vi "remove_invalid_ROI.vi"(8 "error in (no error)":errorcluster, 9 "number of particles":i32, 10 "neighborhood array":T1[](array[typedef]), 11 "Image Pixels in":u8[][](array[numeric])) -> (0 "error out":errorcluster, 2 "ROI array out":T1[](array[typedef]), 3 "Image Pixels out":u8[][](array[numeric]))   [LabVIEW 2010]
uses:
  point_cluster.ctl
panel:
  out "Numeric":i32
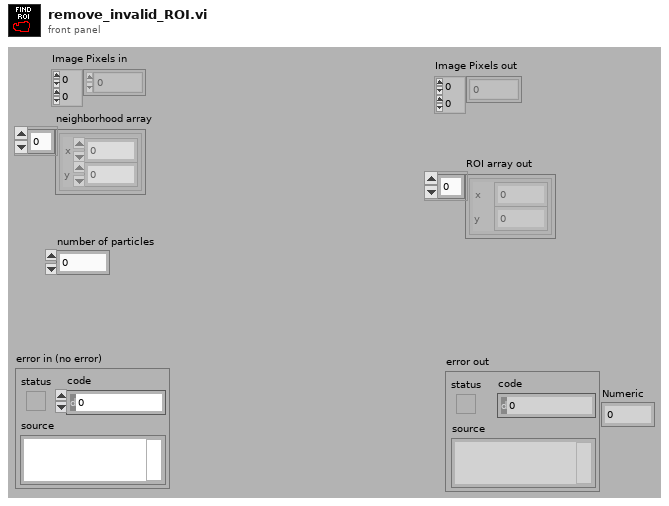
[diagram p1: front panel]
types:
  T1 = typedef "point_cluster.ctl" = cluster{"x":i32, "y":i32}
  T2 = cluster{"[0]":i32, "[1]":i32, "[2]":i32, "[3]":i32, "[4]":i32, "[5]":i32, "[6]":i32, "[7]":i32, "[8]":i32}
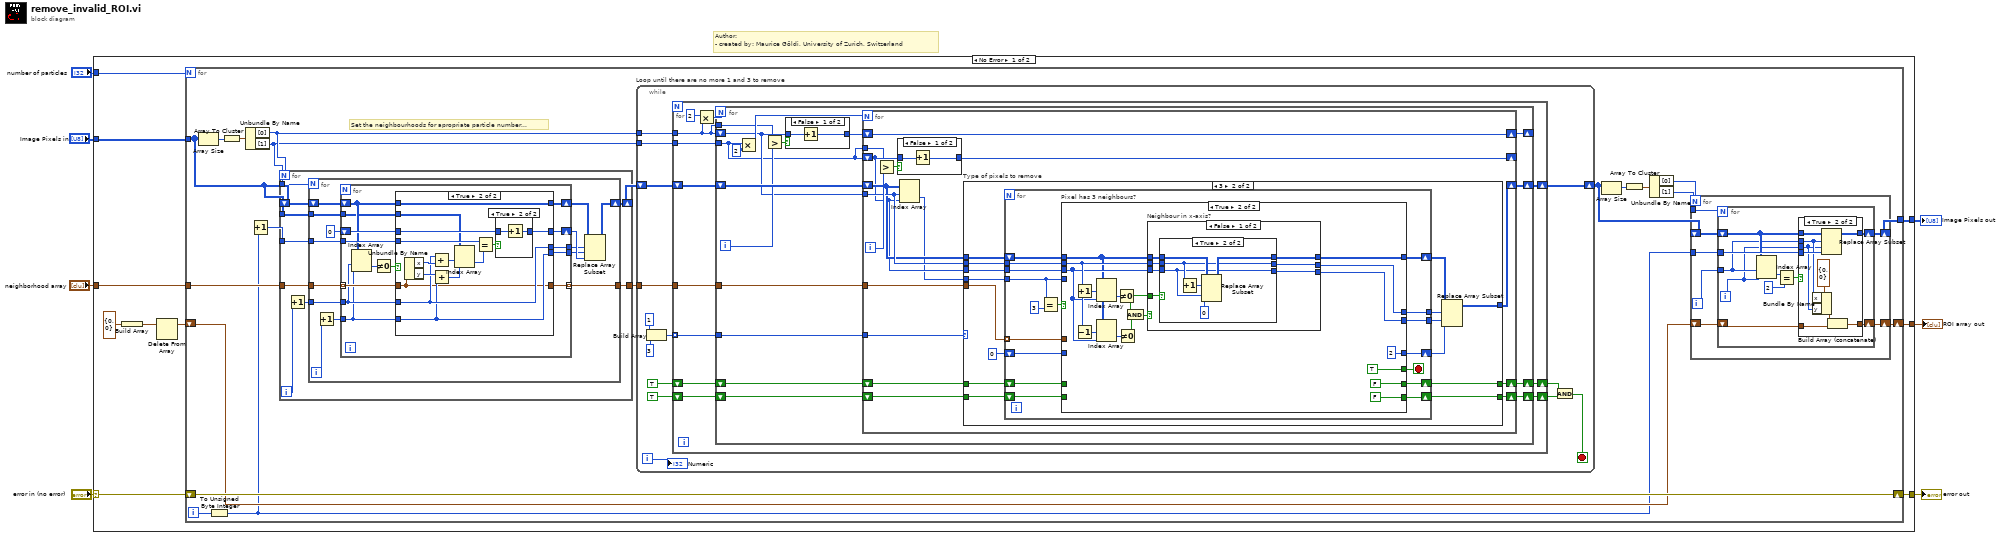
[diagram p0: block diagram]
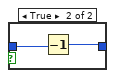
[diagram p5: hidden frame]
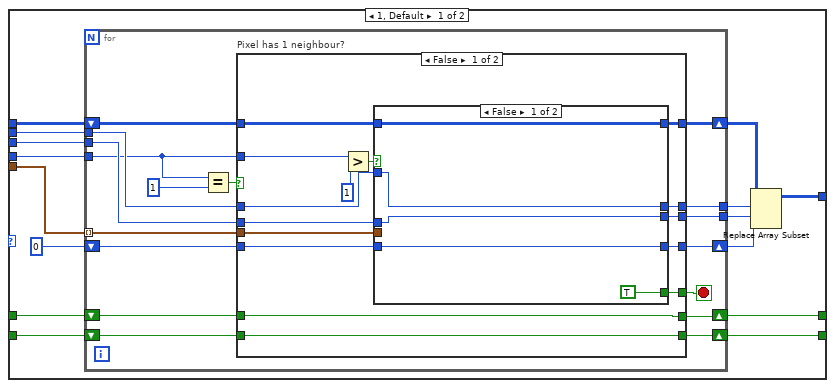
[diagram p6: hidden frame]
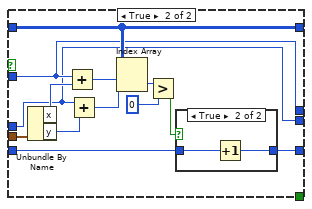
[diagram p7: hidden frame]
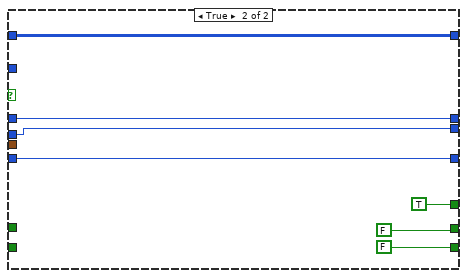
[diagram p9: hidden frame]
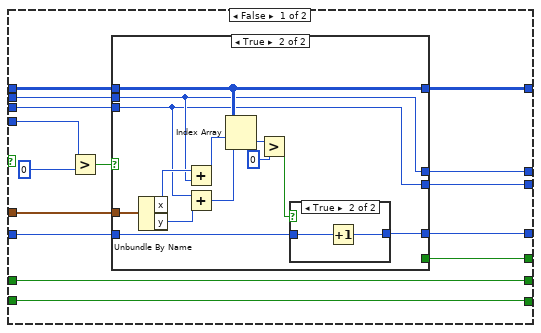
[diagram p10: hidden frame]
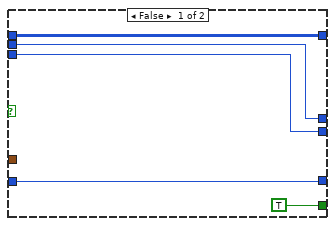
[diagram p11: hidden frame]
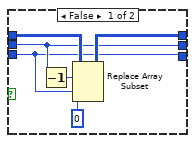
[diagram p13: hidden frame]
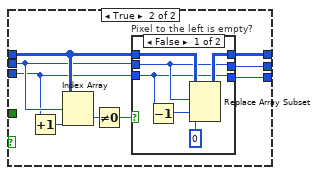
[diagram p14: hidden frame]
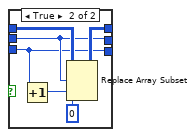
[diagram p15: hidden frame]
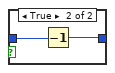
[diagram p16: hidden frame]
diagram:
  # "Author: \n- created by: Maurice Göldi, University of Zurich, Switzerland"
  n1 = case shown="No Error" "error in (no error)" {
    selector: "error in (no error)" -> [w14 w392]
    tunnel: [w13 w392] -> w6
    tunnel: "number of particles" -> [w17 _]
    tunnel: "Image Pixels in" -> [w16 _]
    tunnel: "neighborhood array" -> [w15 _]
    tunnel: [w12 _] -> w2
    tunnel: [w11 _] -> w1
    frame No Error {
      n2 = Build Array(T1 {"x"=0, "y"=0} ("point")) -> (w9:T1[])
      n3 = Delete From Array(array=w9) -> (array with subset deleted=w8:T1[])  [unwired: 2 in, 1 out]
      n4 = for {
        N: w17 -> [_]
        tunnel: w16 -> [w18]
        tunnel: w15 -> [w32]
        shift-right: [w37] -> w13
        shift-left: w14 -> [w37]
        shift-right: [w25] -> w12
        shift-left: w8 -> [w24]
        tunnel: [w23] -> w11
        i -> [w22]
        # "Set the neighbourhoods for apropriate particle number..."
        n5 = Array Size(array=w18) -> (size(s)=w36:i32[])
        n6 = To Unsigned Byte Integer(number=w22) -> (unsigned 8bit integer=w21:u8)
        n7 = Array To Cluster(array=w36) -> (cluster=w35:T2)
        n8 = Unbundle By Name(w35) -> ("[0]"=w34:i32, "[1]"=w33:i32)
        n9 = Increment(x=w21) -> (x+1=w30:u8)
        n10 = for {
          N: w34 -> [_]
          tunnel: w33 -> [w74]
          shift-right: [w72] -> w20
          shift-left: w18 -> [w73]
          tunnel: w32 -> [w71]
          tunnel: [w70] -> w31
          tunnel: w30 -> [w67]
          tunnel: w18 -> [w66]
          i -> [w69]
          n11 = Increment(x=w69) -> (x+1=w68:i32)
          n12 = for {
            N: w74 -> [_]
            shift-right: [w79] -> w72
            shift-left: w73 -> [w86]
            tunnel: [w88] -> w70
            tunnel: w71 -> [w87]
            tunnel: w68 -> [w84]
            tunnel: w67 -> [w82]
            tunnel: w66 -> [w75]
            i -> [w85]
            n13 = Increment(x=w85) -> (x+1=w83:i32)
            n14 = for {
              tunnel: [w90] -> w88 mode=indexing
              tunnel: w87 -> [w102] mode=indexing
              shift-right: [w97] -> w80
              shift-left: w86 -> [w95]
              tunnel: w84 -> [w94]
              tunnel: w83 -> [w93]
              tunnel: w82 -> [w96]
              shift-right: [w100] -> w78
              shift-left: u8 0 -> [w101]
              tunnel: [w99] -> w77
              tunnel: [w98] -> w76
              tunnel: w75 -> [w89]
              n15 = Index Array(array=w95, index (row)=w94, index (col)=w93) -> (element=w91:u8)
              n16 = Not Equal To 0?(x=w91) -> (x != 0?=w92:bool)
              n17 = case shown="True" w92 {
                tunnel: w102 -> [w103 w109]
                tunnel: w95 -> [w104 w110]
                tunnel: w96 -> [_ w115]
                tunnel: w101 -> [w105 w114]
                tunnel: [w105 w113] -> w100
                tunnel: w93 -> [w106 w111]
                tunnel: w94 -> [w107 w112]
                tunnel: [w107 w112] -> w99
                tunnel: [w106 w111] -> w98
                tunnel: [w104 w110] -> w97
                tunnel: [w103 w109] -> w90
                tunnel: w89 -> [_ w108]
                frame False {
                }
                frame True {
                  n18 = Unbundle By Name(w109) -> ("x"=w121:i32, "y"=w120:i32)
                  n19 = Add(x=w112, y=w121) -> (x+y=w119:i32)
                  n20 = Add(x=w120, y=w111) -> (x+y=w118:i32)
                  n21 = Index Array(array=w108, index (row)=w119, index (col)=w118) -> (element=w116:u8)
                  n22 = Equal?(x=w115, y=w116) -> (x = y?=w117:bool)
                  n23 = case shown="True" w117 {
                    tunnel: [w122 w124] -> w113
                    tunnel: w114 -> [w122 w123]
                    frame False {
                    }
                    frame True {
                      n24 = Increment(x=w123) -> (x+1=w124:u8)
                    }
                  }
                }
              }
            }
            n25 = Replace Array Subset(array=w80, new element=w78, index (row)=w77, index (col)=w76) -> (w79:u8[][])
          }
        }
        n26 = while "Loop until there are no more 1 and 3 to remove" {
          tunnel: w31 -> [w138]
          tunnel: w34 -> [w133]
          tunnel: w33 -> [w132]
          shift-right: [w131] -> w19
          shift-left: w20 -> [w130]
          i -> [w129]
          stop <- w127 stop-if-true
          n27 = Build Array(1 ("element"), 3 ("element")) -> (w135:i32[])
          n28 = for {
            tunnel: w138 -> [w147]
            tunnel: w135 -> [w146] mode=indexing
            tunnel: w133 -> [w142]
            tunnel: w132 -> [w144]
            shift-right: [w143] -> w131
            shift-left: w130 -> [w150]
            shift-right: [w139] -> w126
            shift-left: TRUE -> [w145]
            shift-right: [w140] -> w125
            shift-left: TRUE -> [w141]
            n29 = Multiply(x=2, y=w142) -> (x*y=w149:i32)
            n30 = for {
              N: w149 -> [_]
              tunnel: w144 -> [w153]
              shift-right: [w165] -> _
              shift-left: w142 -> [w159]
              shift-right: [w163] -> w143
              shift-left: w150 -> [w164]
              tunnel: w147 -> [w158]
              tunnel: w146 -> [w157]
              shift-right: [w155] -> w139
              shift-left: w145 -> [w156]
              tunnel: w142 -> [w154]
              shift-right: [w151] -> w140
              shift-left: w141 -> [w152]
              i -> [w160]
              n31 = Multiply(x=w153, y=2) -> (x*y=w166:i32)
              n32 = Greater?(x=w154, y=w160) -> (0:w161:bool)
              n33 = case shown="False" w161 {
                tunnel: w159 -> [w169 w170]
                tunnel: [w168 w171] -> w162
                frame False {
                  n34 = Increment(x=w169) -> (x+1=w168:i32)
                }
                frame True {
                  n35 = Decrement(x=w170) -> (x-1=w171:i32)
                }
              }
              n36 = for {
                N: w166 -> [_]
                shift-right: [w187] -> w165
                shift-left: w162 -> [w187]
                shift-right: [w186] -> _
                shift-left: w153 -> [w179]
                shift-right: [w177] -> w163
                shift-left: w164 -> [w180]
                tunnel: w159 -> [w181]
                tunnel: w158 -> [w183]
                tunnel: w157 -> [w182]
                shift-right: [w175] -> w155
                shift-left: w156 -> [w176]
                tunnel: w153 -> [w174]
                shift-right: [w172] -> w151
                shift-left: w152 -> [w173]
                i -> [w184]
                n37 = Greater?(x=w174, y=w184) -> (0:w185:bool)
                n38 = case shown="False" w185 {
                  tunnel: w179 -> [w389 w390]
                  tunnel: [w388 w391] -> w186
                  frame False {
                    n39 = Increment(x=w389) -> (x+1=w388:i32)
                  }
                  frame True {
                    n40 = Decrement(x=w390) -> (x-1=w391:i32)
                  }
                }
                n41 = Index Array(array=w180, index (row)=w181, index (col)=w179) -> (element=w178:u8)
                n42 = case "Type of pixels to remove" shown="3" w182 {
                  tunnel: w183 -> [w202 w273]
                  tunnel: w181 -> [w201 w276]
                  tunnel: w179 -> [w200 w275]
                  tunnel: w180 -> [w199 w277]
                  tunnel: w178 -> [w198 w274]
                  tunnel: [w192 w271] -> w177
                  tunnel: w176 -> [w190 w267]
                  tunnel: [w189 w266] -> w175
                  tunnel: w173 -> [w191 w264]
                  tunnel: [w188 w263] -> w172
                  frame 1, Default {
                    n43 = for {
                      tunnel: w202 -> [w213] mode=indexing
                      tunnel: w201 -> [w217]
                      tunnel: w200 -> [w216]
                      shift-right: [w210] -> w195
                      shift-left: w199 -> [w214]
                      tunnel: w198 -> [w215]
                      shift-right: [w211] -> w196
                      shift-left: u8 0 -> [w212]
                      tunnel: [w209] -> w194
                      tunnel: [w208] -> w193
                      shift-right: [w206] -> w188
                      shift-left: w191 -> [w205]
                      shift-right: [w203] -> w189
                      shift-left: w190 -> [w204]
                      stop <- w207 stop-if-true
                      n44 = Equal?(x=w215, y=u8 1) -> (x = y?=w218:bool)
                      n45 = case "Pixel has 1 neighbour?" shown="False" w218 {
                        tunnel: w214 -> [w226 w261]
                        tunnel: w217 -> [w230 w260]
                        tunnel: w216 -> [w229 w259]
                        tunnel: w215 -> [w233 _]
                        tunnel: w213 -> [w231 _]
                        tunnel: w212 -> [w228 w262]
                        tunnel: [w227 w262] -> w211
                        tunnel: [w225 w261] -> w210
                        tunnel: [w224 w260] -> w209
                        tunnel: [w223 w259] -> w208
                        tunnel: [w222 TRUE] -> w207
                        tunnel: [w220 FALSE] -> w206
                        tunnel: w205 -> [w220 _]
                        tunnel: [w221 FALSE] -> w203
                        tunnel: w204 -> [w221 _]
                        frame False {
                          n46 = Greater?(x=w233, y=u8 1) -> (0:w234:bool)
                          n47 = case shown="False" w234 {
                            tunnel: w226 -> [w238 w244]
                            tunnel: w231 -> [_ w250]
                            tunnel: w230 -> [w237 w243]
                            tunnel: w229 -> [w236 w242]
                            tunnel: w228 -> [w239 w246]
                            tunnel: [w239 w245] -> w227
                            tunnel: [w238 w244] -> w225
                            tunnel: [w237 w243] -> w224
                            tunnel: [w236 w242] -> w223
                            tunnel: [TRUE _] -> w222
                            frame False {
                            }
                            frame True {
                              n48 = Unbundle By Name(w250) -> ("x"=w251:i32, "y"=w252:i32)
                              n49 = Add(x=w243, y=w251) -> (x+y=w241:i32)
                              n50 = Add(x=w242, y=w252) -> (x+y=w240:i32)
                              n51 = Index Array(array=w244, index (row)=w241, index (col)=w240) -> (element=w249:u8)
                              n52 = Greater?(x=w249, y=u8 0) -> (0:w247:bool)
                              n53 = case shown="True" w247 {
                                tunnel: w246 -> [w253 w255]
                                tunnel: [w253 w254] -> w245
                                frame False {
                                }
                                frame True {
                                n54 = Increment(x=w255) -> (x+1=w254:u8)
                                }
                              }
                            }
                          }
                        }
                        frame True {
                        }
                      }
                    }
                    n55 = Replace Array Subset(array=w195, new element=w196, index (row)=w194, index (col)=w193) -> (w192:u8[][])
                  }
                  frame 3 {
                    n56 = for {
                      tunnel: w276 -> [w291]
                      tunnel: w275 -> [w290]
                      tunnel: w274 -> [w282]
                      tunnel: w273 -> [w289] mode=indexing
                      shift-right: [w286] -> w265
                      shift-left: w277 -> [w294]
                      shift-right: [w287] -> w268
                      shift-left: u8 0 -> [w288]
                      tunnel: [w285] -> w270
                      tunnel: [w284] -> w269
                      shift-right: [w280] -> w266
                      shift-left: w267 -> [w281]
                      shift-right: [w278] -> w263
                      shift-left: w264 -> [w279]
                      stop <- w283 stop-if-true
                      n57 = Equal?(x=w282, y=u8 3) -> (x = y?=w293:bool)
                      n58 = case "Pixel has 3 neighbours?" shown="True" w293 {
                        tunnel: w294 -> [w307 w336]
                        tunnel: w291 -> [w305 w338]
                        tunnel: w290 -> [w304 w337]
                        tunnel: w289 -> [w306 _]
                        tunnel: w288 -> [w308 _]
                        tunnel: [w309 u8 2] -> w287
                        tunnel: [w303 w335] -> w286
                        tunnel: [w302 w332] -> w285
                        tunnel: [w301 w331] -> w284
                        tunnel: [w297 TRUE] -> w283
                        tunnel: w282 -> [w298 _]
                        tunnel: w281 -> [w295 _]
                        tunnel: [w295 FALSE] -> w280
                        tunnel: w279 -> [w296 _]
                        tunnel: [w296 FALSE] -> w278
                        frame False {
                          n59 = Greater?(x=w298, y=u8 0) -> (0:w300:bool)
                          n60 = case shown="True" w300 {
                            tunnel: [w314 w327] -> w309
                            tunnel: w308 -> [w314 w326]
                            tunnel: w307 -> [w310 w322]
                            tunnel: w306 -> [_ w325]
                            tunnel: w305 -> [w312 w318]
                            tunnel: w304 -> [w313 w317]
                            tunnel: [w310 w322] -> w303
                            tunnel: [w313 w317] -> w301
                            tunnel: [w312 w318] -> w302
                            tunnel: [TRUE _] -> w297
                            frame False {
                            }
                            frame True {
                              n61 = Unbundle By Name(w325) -> ("x"=w323:i32, "y"=w324:i32)
                              n62 = Add(x=w323, y=w318) -> (x+y=w316:i32)
                              n63 = Add(x=w317, y=w324) -> (x+y=w315:i32)
                              n64 = Index Array(array=w322, index (row)=w316, index (col)=w315) -> (element=w321:u8)
                              n65 = Greater?(x=w321, y=u8 0) -> (0:w319:bool)
                              n66 = case shown="True" w319 {
                                tunnel: [w328 w330] -> w327
                                tunnel: w326 -> [w328 w329]
                                frame False {
                                }
                                frame True {
                                n67 = Increment(x=w329) -> (x+1=w330:u8)
                                }
                              }
                            }
                          }
                        }
                        frame True {
                          n68 = Increment(x=w338) -> (x+1=w343:i32)
                          n69 = Decrement(x=w338) -> (x-1=w344:i32)
                          n70 = Index Array(array=w336, index (row)=w343, index (col)=w337) -> (element=w342:u8)
                          n71 = Index Array(array=w336, index (row)=w344, index (col)=w337) -> (element=w341:u8)
                          n72 = Not Equal To 0?(x=w342) -> (x != 0?=w333:bool)
                          n73 = Not Equal To 0?(x=w341) -> (x != 0?=w340:bool)
                          n74 = And(x=w333, y=w340) -> (x .and. y?=w339:bool)
                          n75 = case "Neighbour in x-axis?" shown="False" w339 {
                            tunnel: w338 -> [w352 w370]
                            tunnel: w337 -> [w351 w369]
                            tunnel: w336 -> [w353 w372]
                            tunnel: [w350 w371] -> w335
                            tunnel: [w349 w368] -> w332
                            tunnel: [w348 w367] -> w331
                            tunnel: w333 -> [w354 _]
                            frame False {
                              n76 = case shown="True" w354 {
                                tunnel: w353 -> [w359 w365]
                                tunnel: w352 -> [w356 w362]
                                tunnel: w351 -> [w355 w361]
                                tunnel: [w358 w364] -> w350
                                tunnel: [w356 w362] -> w349
                                tunnel: [w355 w361] -> w348
                                frame False {
                                n77 = Decrement(x=w356) -> (x-1=w357:i32)
                                n78 = Replace Array Subset(array=w359, new element=u8 0 ("new element/subarray"), index (row)=w357, index (col)=w355) -> (w358:u8[][])
                                }
                                frame True {
                                n79 = Increment(x=w362) -> (x+1=w366:i32)
                                n80 = Replace Array Subset(array=w365, new element=u8 0 ("new element/subarray"), index (row)=w366, index (col)=w361) -> (w364:u8[][])
                                }
                              }
                            }
                            frame True {
                              n81 = Increment(x=w369) -> (x+1=w374:i32)
                              n82 = Index Array(array=w372, index (row)=w370, index (col)=w374) -> (element=w375:u8)
                              n83 = Not Equal To 0?(x=w375) -> (x != 0?=w373:bool)
                              n84 = case "Pixel to the left is empty?" shown="False" w373 {
                                tunnel: w372 -> [w379 w386]
                                tunnel: [w378 w385] -> w371
                                tunnel: [w377 w383] -> w368
                                tunnel: w370 -> [w377 w383]
                                tunnel: [w376 w382] -> w367
                                tunnel: w369 -> [w376 w382]
                                frame False {
                                n85 = Decrement(x=w376) -> (x-1=w380:i32)
                                n86 = Replace Array Subset(array=w379, new element=u8 0 ("new element/subarray"), index (row)=w377, index (col)=w380) -> (w378:u8[][])
                                }
                                frame True {
                                n87 = Increment(x=w382) -> (x+1=w387:i32)
                                n88 = Replace Array Subset(array=w386, new element=u8 0 ("new element/subarray"), index (row)=w383, index (col)=w387) -> (w385:u8[][])
                                }
                              }
                            }
                          }
                        }
                      }
                    }
                    n89 = Replace Array Subset(array=w265, new element=w268, index (row)=w270, index (col)=w269) -> (w271:u8[][])
                  }
                }
              }
            }
          }
          n90 = And(x=w126, y=w125) -> (x .and. y?=w127:bool)
          "Numeric" <- w129
        }
        n91 = Array Size(array=w19) -> (size(s)=w29:i32[])
        n92 = Array To Cluster(array=w29) -> (cluster=w28:T2)
        n93 = Unbundle By Name(w28) -> ("[0]"=w27:i32, "[1]"=w26:i32)
        n94 = for {
          N: w27 -> [_]
          tunnel: w26 -> [w44]
          tunnel: w21 -> [w41]
          shift-right: [w42] -> w23
          shift-left: w19 -> [w43]
          shift-right: [w40] -> w25
          shift-left: w24 -> [w39]
          i -> [w38]
          n95 = for {
            N: w44 -> [_]
            shift-right: [w54] -> w42
            shift-left: w43 -> [w51]
            tunnel: w38 -> [w50]
            tunnel: w41 -> [w53]
            shift-right: [w47] -> w40
            shift-left: w39 -> [w46]
            i -> [w45]
            n96 = Index Array(array=w51, index (row)=w50, index (col)=w45) -> (element=w52:u8)
            n97 = Equal?(x=w52, y=u8 2) -> (x = y?=w49:bool)
            n98 = case shown="True" w49 {
              tunnel: w51 -> [w56 w65]
              tunnel: [w56 w64] -> w54
              tunnel: w50 -> [_ w60]
              tunnel: w45 -> [_ w59]
              tunnel: w53 -> [_ w63]
              tunnel: [w55 w58] -> w47
              tunnel: w46 -> [w55 w57]
              frame False {
              }
              frame True {
                n99 = Bundle By Name(cluster=T1 {"x"=0, "y"=0} ("point"), "x"=w60, "y"=w59) -> (w61:T1)
                n100 = Replace Array Subset(array=w65, new element=w63, index (row)=w60, index (col)=w59) -> (w64:u8[][])
                n101 = Build Array (concatenate)(w61, w57) -> (w58:T1[])
              }
            }
          }
        }
      }
    }
    frame Error {
    }
  }
  "error out" <- w6
  "Image Pixels out" <- w1
  "ROI array out" <- w2
